vi "Position_GRBL.vi"() -> ()   [LabVIEW 2014, in "GRBLMotionCore.lvlib"]
uses:
  <instrlib>/GRBL/GRBLMotionCore.lvlib
panel:
  in  "Grbl-State":i32(ring) items=["Idle", "Queue", "Run", "Hold", "Home", "Alarm", "Check", "InternalError"]
  in  "tickcount_pos":u32
  out "Moving(Grbl)":bool
  in  "Position(Grbl)":dbl[](array[numeric]) caption="Position" format="%.4f"
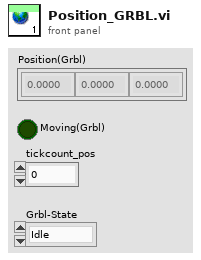
[diagram p1: front panel]
diagram:
